vi "Volt Reader Trigger10.vi"() -> ()   [LabVIEW 2014]
uses:
  Enum State Machine Typedef.ctl
  <vilib>/Utility/error.llb/DialogType.ctl
  <vilib>/_DAQmxBase/Internals/DAQmxBase Create Channel (AI-Voltage-Basic).vi
  <vilib>/_DAQmxBase/Internals/DAQmxBase Timing (Sample Clock).vi
  <vilib>/measure/mamon.llb/Trigger Detection for 1 Channel.vi
  <vilib>/_DAQmxBase/Internals/DAQmxBase Read (Analog 2D DBL NChan NSamp).vi
  <vilib>/measure/NI_MAPro.lvlib
panel:
  out "Waveform Raw":waveform(dbl)(graph)
  in  "Offset (percent of buffer)":dbl(knob) scale=-50.0..50.0
  in  "Timeout (in iterations)":i16
  out "State":T1
  out "Waveform Graph":waveform(dbl)(graph)
  in  "Buffer (Seconds)":dbl
  out "Threshold":dbl
  in  "units":i32(ring)=10348 items=["Volts"=10348, "From Custom Scale"=10065]
  in  "stop":bool
  in  "physical channels":tag
  in  "maximum value":dbl=5.0 format="%0.2f"
  in  "minimum value":dbl=-5.0 format="%0.2f"
  in  "rate":i32=1000 caption="Sample Rate"
  # "The inputs above MUST BE\nPreset before running"
  # "NOTE: Just change the Y axis value"
  # "Make Sure that Buffer does not equal 0"
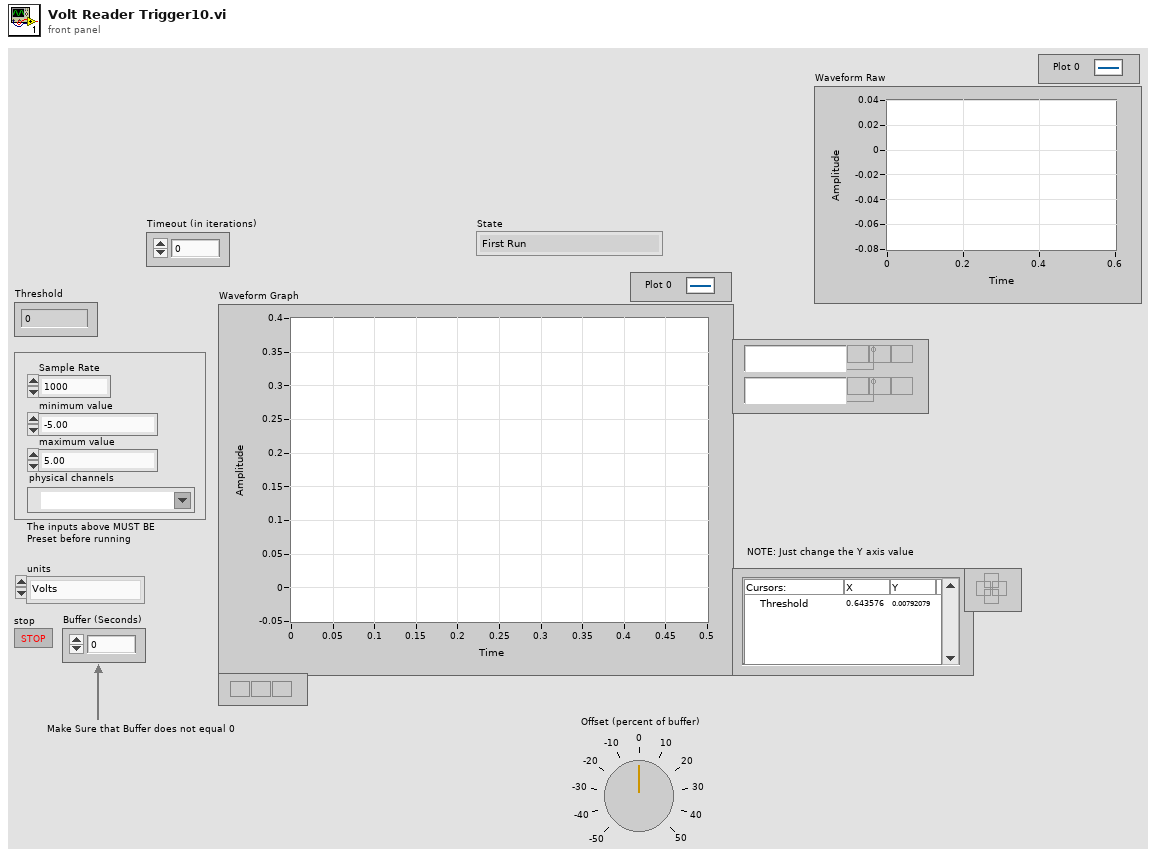
[diagram p1: front panel]
types:
  T1 = typedef "Enum State Machine Typedef.ctl" = enum16{"First Run", "Gather and Edit Data", "Find Max with Gather Data", "Trigger Occured", "Found the Max", "Just Displayed", "The Max is in the Middle", "Base State", "Timeout"}
  T2 = typedef "DialogType.ctl" = u16
  T3 = typedef "LVCursorListTypeDef.ctl" = cluster{"Name":string, "Color":u32, "Style":u8, "Point Style":u8, "Name Visible":bool, "Allow Drag":bool, "Cursor Mode":u32, "Plot":i32, "Index":i32, "Position":cluster{"X":dbl, "Y":dbl}, "X Scale":u32, "Y Scale":u32, "Watch Plots":i32[], "Watch All Plots":bool, "Plot Area":i32, "Label Offset":cluster{"X":dbl, "Y":dbl}}[]
  T4 = cluster{"Name":string, "Color":u32, "Style":u8, "Point Style":u8, "Name Visible":bool, "Allow Drag":bool, "Cursor Mode":u32, "Plot":i32, "Index":i32, "Position":cluster{"X":dbl, "Y":dbl}, "X Scale":u32, "Y Scale":u32, "Watch Plots":i32[], "Watch All Plots":bool, "Plot Area":i32, "Label Offset":cluster{"X":dbl, "Y":dbl}}
  T5 = enum16{"In the Center Range", "Before the Center Range", "After the Center Range"}
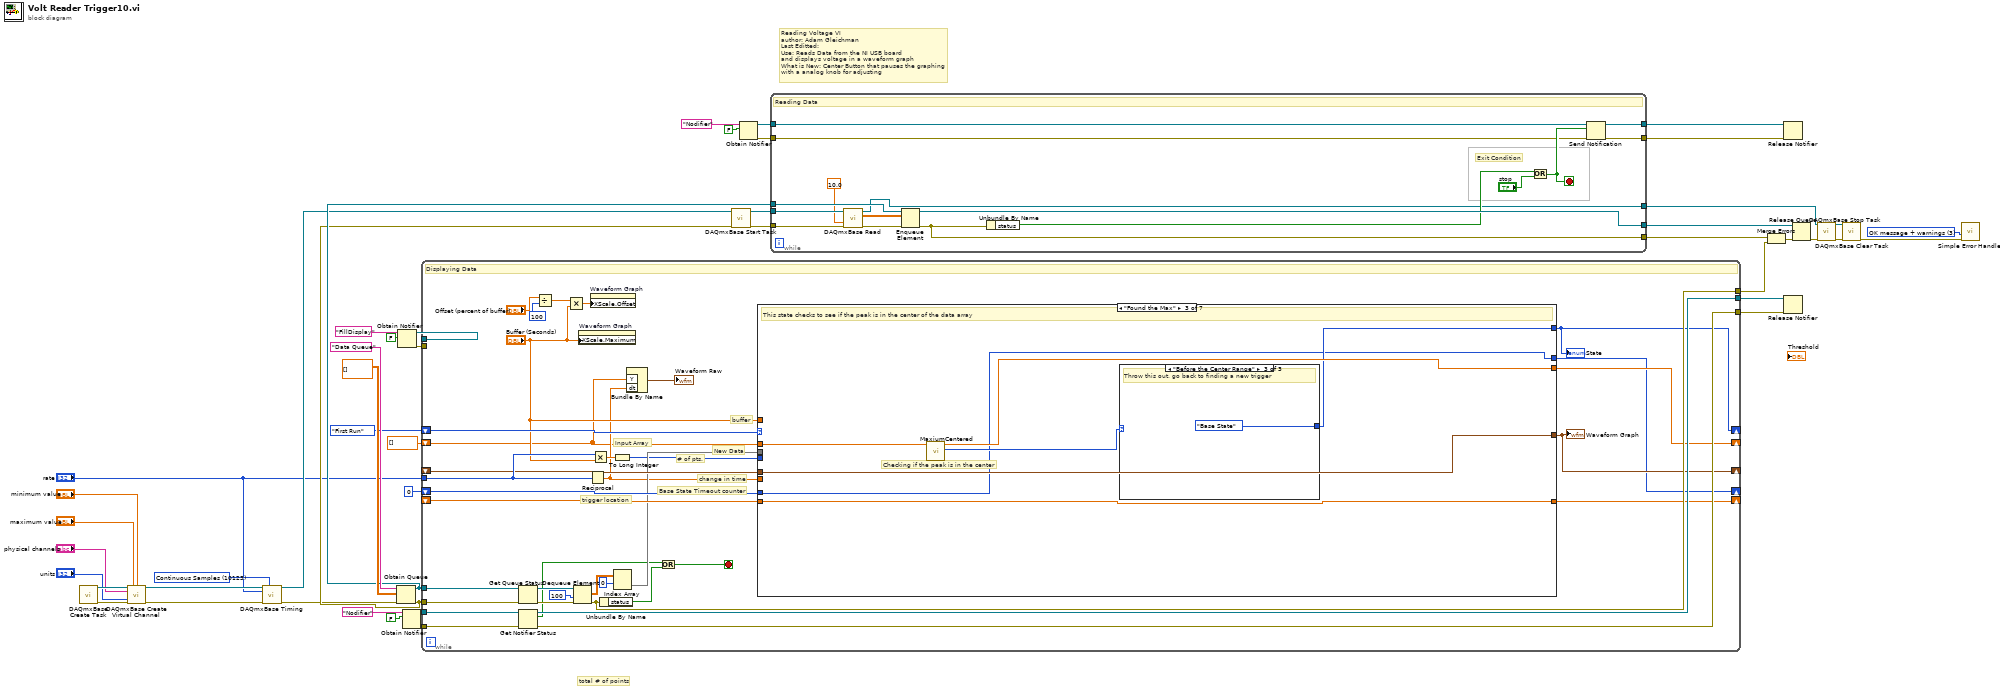
[diagram p0: block diagram]
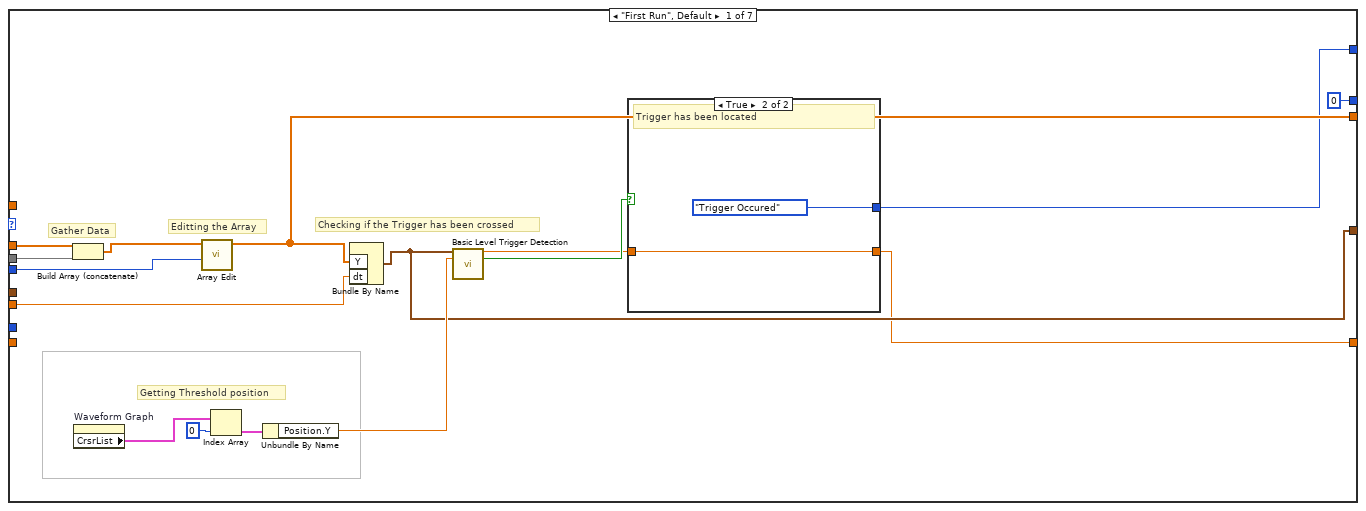
[diagram p2: hidden frame]
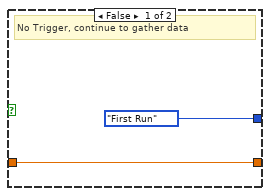
[diagram p3: hidden frame]
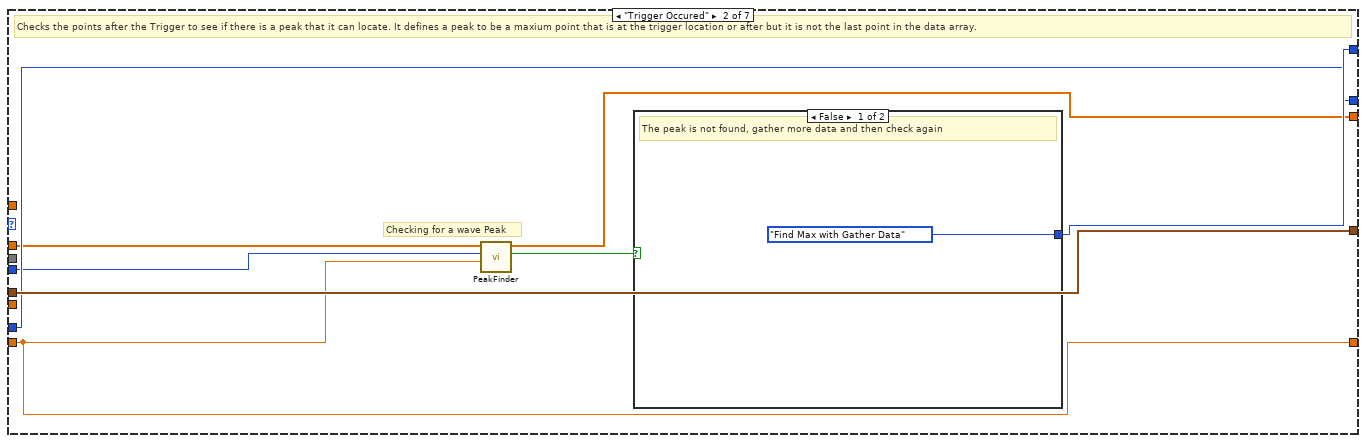
[diagram p4: hidden frame]
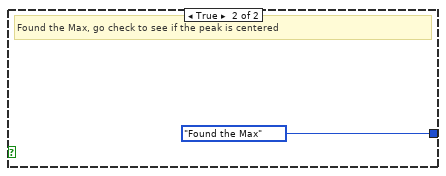
[diagram p5: hidden frame]
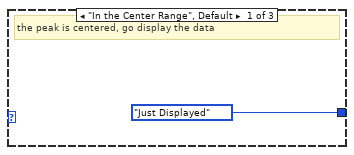
[diagram p6: hidden frame]
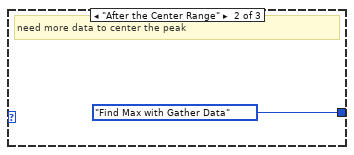
[diagram p7: hidden frame]
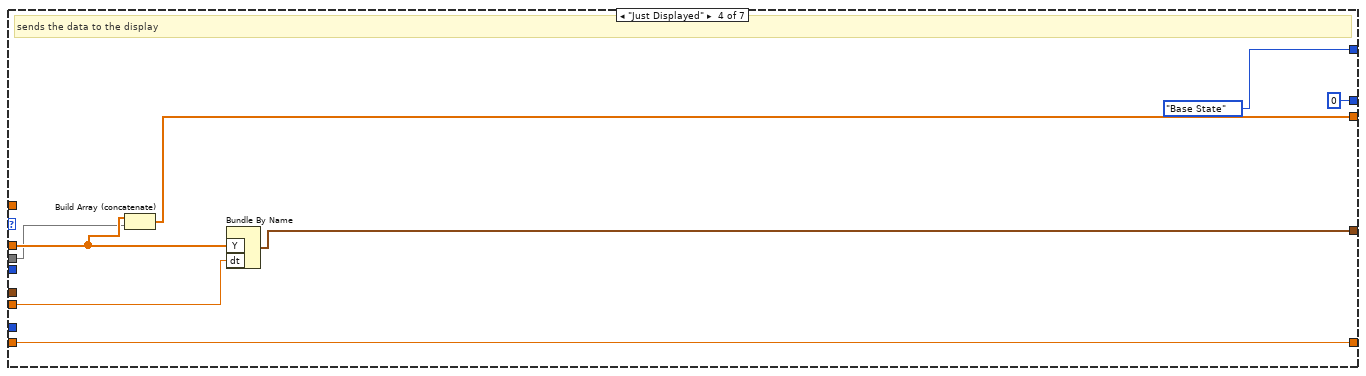
[diagram p8: hidden frame]
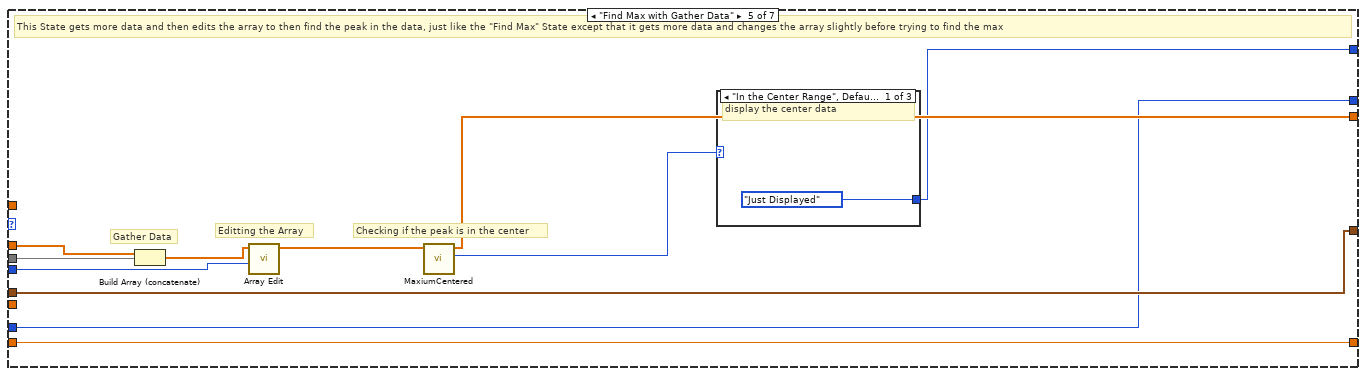
[diagram p9: hidden frame]
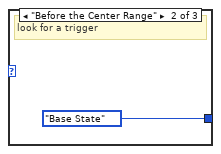
[diagram p10: hidden frame]
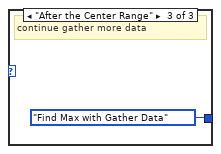
[diagram p11: hidden frame]
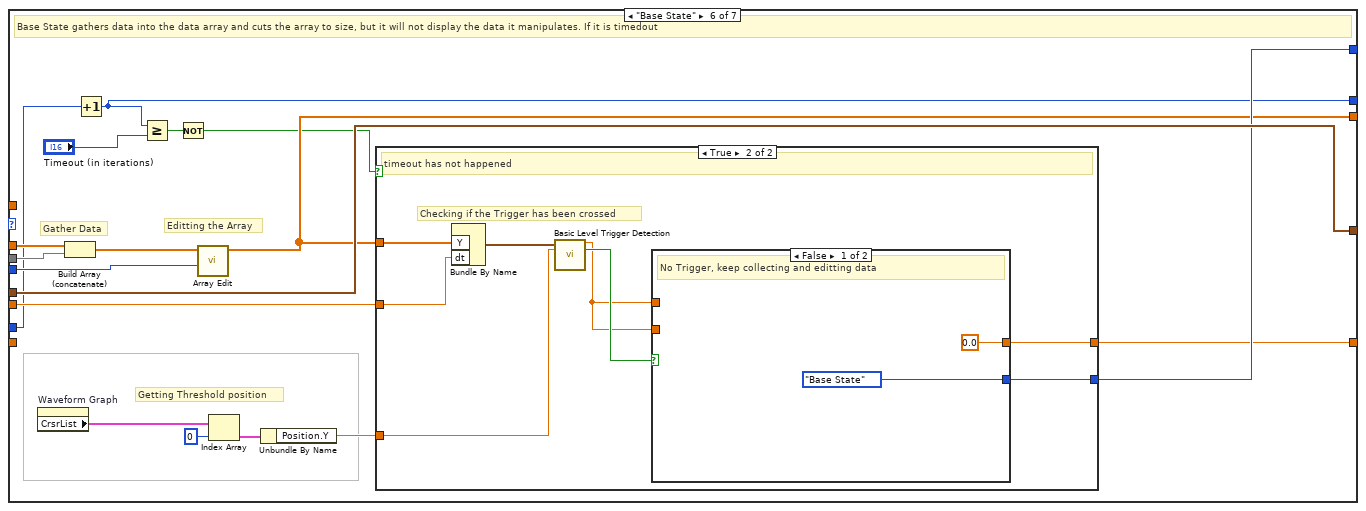
[diagram p12: hidden frame]
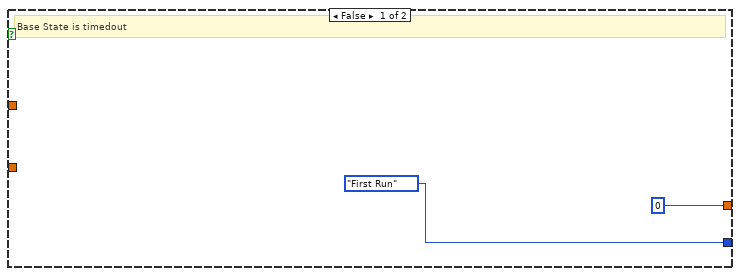
[diagram p13: hidden frame]
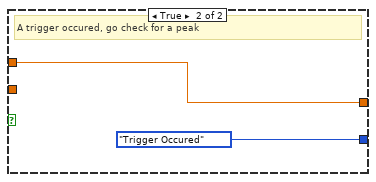
[diagram p14: hidden frame]
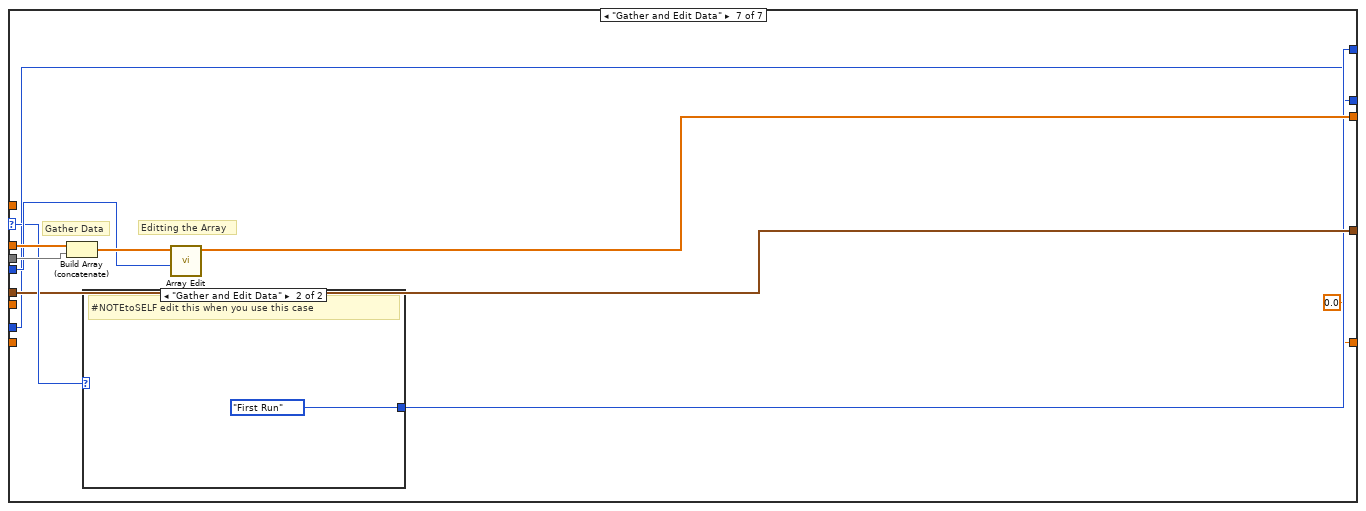
[diagram p15: hidden frame]
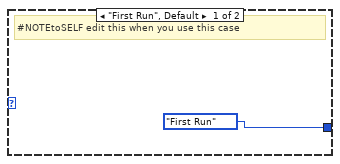
[diagram p16: hidden frame]
diagram:
  w24 = 10123 items=["Finite Samples"=10178, "Continuous Samples"=10123, "Hardware Timed Single Point"=12522] ("sample mode")
  w26 = T2 3 items=["no dialog", "OK message", "continue or stop message", "OK message + warnings", "continue/stop + warnings"] ("type of dialog (OK msg:1)")
  # "total # of points"
  # "Reading Voltage VI\nauthor: Adam Gleichman\nLast Editted: \nUse: Reads Data from the NI USB board\nand displays voltage in a waveform graph\nWhat is New: Center Button that pauses the graphing\nwith a analog knob for adjusting"
  n1 = call <vilib>:"DAQmxBase Create Task.vi"() -> ("task out"=w46:refnum<k21>, "error out"=w45:errorcluster)  [unwired: 5 in, 9 out]
  n2 = call-poly <vilib>:"DAQmxBase Create Virtual Channel.vi"("task in"=w46, "maximum value"="maximum value", "minimum value"="minimum value", "physical channels"="physical channels", "units"="units", "error in"=w45) -> ("task out"=w43:refnum<k21>, "error out"=w44:errorcluster)  [unwired: 3 in, 5 out]
  n3 = call-poly <vilib>:"DAQmxBase Timing.vi"("task/channels in"=w43, "sample mode"=w24, "rate"="rate", "error in"=w44) -> ("task out"=w12:refnum<k21>, "error out"=w11:errorcluster)  [unwired: 3 in, 7 out]
  n4 = Obtain Queue(name (unnamed)="Data Queue", element data type=dbl[][] [] ("data"), error in (no error)=w11) -> (queue out=w33:refnum<queue>, error out=w32:errorcluster)  [unwired: 2 in, 1 out]
  n5 = Obtain Notifier(name (unnamed)="FillDisplay", notification data type=FALSE) -> (notifier out=w8:refnum<notifier>, error out=w7:errorcluster)  [unwired: 2 in, 1 out]
  n6 = Obtain Notifier(name (unnamed)="Nodifier", notification data type=FALSE) -> (notifier out=w17:refnum<notifier>, error out=w15:errorcluster)  [unwired: 2 in, 1 out]
  n7 = while {
    tunnel: w33 -> [w83]
    tunnel: w32 -> [w74]
    tunnel: [w81] -> w31
    tunnel: w17 -> [w79]
    tunnel: w15 -> [w78]
    tunnel: [w77] -> w13
    tunnel: [w76] -> w14
    tunnel: "rate" -> [w70]
    shift-right: [w65] -> _
    shift-left: dbl[] [] -> [w49]
    tunnel: w8 -> [_]
    tunnel: w7 -> [_]
    shift-right: [w64] -> _
    shift-left: Enum_State_Machine_Typedef."First Run" -> [w67]
    shift-right: [w66] -> _
    shift-left: _ -> [w68]
    shift-right: [w62] -> _
    shift-left: 0 -> [w63]
    shift-right: [w61] -> _
    shift-left: _ -> [w60]
    stop <- w80 stop-if-true
    # "trigger location"
    # "change in time"
    # "buffer"
    # "Base State Timeout counter"
    # "New Data"
    # "Input Array"
    # "# of pts."
    # "Displaying Data"
    n8 = Get Queue Status(queue=w83, error in (no error)=w74) -> (queue out=w75:refnum<queue>, error out=w73:errorcluster)  [unwired: 1 in, 6 out]
    n9 = Get Notifier Status(notifier=w79, error in (no error)=w78) -> (notifier out=w77:refnum<notifier>, current notification=w51:bool, error out=w76:errorcluster)  [unwired: 2 out]
    n10 = Divide(x="Offset (percent of buffer)", y=100) -> (x/y=w54:dbl)
    n11 = Multiply(x=w54, y="Buffer (Seconds)") -> (x*y=w53:dbl)
    n12 = Dequeue Element(queue=w75, timeout in ms (-1)=100, error in (no error)=w73) -> (element=w71:dbl[][], error out=w81:errorcluster)  [unwired: 2 out]
    n13 = property on="Waveform Graph" class="WFGraph (strict)"("XScale.Maximum"="Buffer (Seconds)") -> ()  [unwired: 2 in, 2 out]
    n14 = Reciprocal(x=w70) -> (1/x=w50:dbl)
    n15 = property on="Waveform Graph" class="WFGraph (strict)"("XScale.Offset"=w53) -> ()  [unwired: 2 in, 2 out]
    n16 = Multiply(x=w70, y="Buffer (Seconds)") -> (x*y=w69:dbl)
    n17 = Unbundle By Name(w81) -> ("status"=w52:bool)
    n18 = To Long Integer(number=w69) -> (32bit integer=w58:i32)
    n19 = Index Array(array=w71, index (row)=0 ("index")) -> (element=w59:dbl[])  [unwired: 1 in]
    n20 = Bundle By Name("Y"=w49, "dt"=w50) -> (→"Waveform Raw":waveform(dbl))  [unwired: 1 in]
    n21 = Or(x=w51, y=w52) -> (x .or. y?=w80:bool)
    n22 = case shown="\"Found the Max\"" w67 {
      selector: w67 -> [_ _ _ _ _ _ w183]
      tunnel: w49 -> [w99 w108 w120 w130 w142 w163 w187]
      tunnel: w59 -> [w98 _ _ w129 w141 w162 w186]
      tunnel: w50 -> [w92 _ _ w131 _ w156 _]
      tunnel: w58 -> [w96 w105 _ _ w139 w160 w184]
      tunnel: [w89 w111 w116 w127 w134 w155 w181] -> w66
      tunnel: w68 -> [_ w111 w116 _ w134 w155 w181]
      tunnel: "Buffer (Seconds)" -> [_ _ _ _ _ _ _]
      tunnel: [w88 w107 w119 w128 w136 w153 w182] -> w65
      tunnel: [w87 w110 w117 Enum_State_Machine_Typedef."Base State" w135 w154 w180] -> w64
      tunnel: w63 -> [_ w109 w114 _ w133 w151 w179]
      tunnel: [0 w109 w114 0 w133 w147 w179] -> w62
      tunnel: [w85 w104 w115 w125 w132 w146 0.0 ("trigger location")] -> w61
      tunnel: w60 -> [_ w104 w115 w125 w132 _ _]
      frame "First Run", Default {
        # "Checking if the Trigger has been crossed"
        # "Getting Threshold position"
        # "Editting the Array"
        # "Gather Data"
        n23 = Build Array (concatenate)(w99, w98) -> (w97:dbl[])
        n24 = property on="Waveform Graph" class="WFGraph (strict)"() -> ("CrsrList"=w94:T3)  [unwired: 2 in, 2 out]
        n25 = call "Array Edit.vi"("Number of Points"=w96, "Y-values"=w97) -> ("Editted Y Values"=w88:dbl[])  [unwired: 9 in]
        n26 = Index Array(array=w94, index=0) -> (element=w95:T4)
        n27 = Unbundle By Name(w95) -> ("Position.Y"=w91:dbl)
        n28 = Bundle By Name("Y"=w88, "dt"=w92) -> (w89:waveform(dbl))  [unwired: 1 in]
        n29 = call-poly <vilib>:"Basic Level Trigger Detection.vi"("signal in"=w89, "level"=w91) -> ("trigger location"=w86:dbl, "trigger detected?"=w90:bool)  [unwired: 11 in, 1 out]
        n30 = case shown="True" w90 {
          tunnel: [Enum_State_Machine_Typedef."First Run" Enum_State_Machine_Typedef."Trigger Occured"] -> w87
          tunnel: w86 -> [w100 w102]
          tunnel: [w100 w102] -> w85
          frame False {
            # "No Trigger, continue to gather data"
          }
          frame True {
            # "Trigger has been located"
          }
        }
      }
      frame "Trigger Occured" {
        # "Checking for a wave Peak"
        # "Checks the points after the Trigger to see if there is a peak that it can locate. It defines a peak to be a maxium point that is at the trigger location or after but it is not the last point in the data array."
        n31 = call "PeakFinder.vi"("Trigger location"=w104, "Number of Points"=w105, "Input Y values"=w108) -> ("peak?"=w106:bool, "Input Y values"=w107:dbl[])  [unwired: 7 in]
        n32 = case shown="False" w106 {
          tunnel: [Enum_State_Machine_Typedef."Find Max with Gather Data" Enum_State_Machine_Typedef."Found the Max"] -> w110
          frame False {
            # "The peak is not found, gather more data and then check again"
          }
          frame True {
            # "Found the Max, go check to see if the peak is centered"
          }
        }
      }
      frame "Found the Max" {
        # "Checking if the peak is in the center"
        # "This state checks to see if the peak is in the center of the data array"
        n33 = call "MaxiumCentered.vi"("Input Y Values"=w120) -> ("State output"=w118:T5, "Output Y Values"=w119:dbl[])  [unwired: 9 in]
        n34 = case shown="\"Before the Center Range\"" w118 {
          tunnel: [Enum_State_Machine_Typedef."Just Displayed" Enum_State_Machine_Typedef."Find Max with Gather Data" Enum_State_Machine_Typedef."Base State"] -> w117
          frame "In the Center Range", Default {
            # "the peak is centered, go display the data"
          }
          frame "After the Center Range" {
            # "need more data to center the peak"
          }
          frame "Before the Center Range" {
            # "Throw this out, go back to finding a new trigger"
          }
        }
      }
      frame "Just Displayed" {
        # "sends the data to the display"
        n35 = Build Array (concatenate)(w130, w129) -> (w128:dbl[])
        n36 = Bundle By Name("Y"=w130, "dt"=w131) -> (w127:waveform(dbl))  [unwired: 1 in]
      }
      frame "Find Max with Gather Data" {
        # "Editting the Array"
        # "Gather Data"
        # "Checking if the peak is in the center"
        # "This State gets more data and then edits the array to then find the peak in the data, just like the \"Find Max\" State except that it gets more data and changes the array slightly before trying to find the max"
        n37 = Build Array (concatenate)(w142, w141) -> (w140:dbl[])
        n38 = call "Array Edit.vi"("Number of Points"=w139, "Y-values"=w140) -> ("Editted Y Values"=w138:dbl[])  [unwired: 9 in]
        n39 = call "MaxiumCentered.vi"("Input Y Values"=w138) -> ("State output"=w137:T5, "Output Y Values"=w136:dbl[])  [unwired: 9 in]
        n40 = case shown="\"In the Center Range\", Default" w137 {
          tunnel: [Enum_State_Machine_Typedef."Just Displayed" Enum_State_Machine_Typedef."Base State" Enum_State_Machine_Typedef."Find Max with Gather Data"] -> w135
          frame "In the Center Range", Default {
            # "display the center data"
          }
          frame "Before the Center Range" {
            # "look for a trigger"
          }
          frame "After the Center Range" {
            # "continue gather more data"
          }
        }
      }
      frame "Base State" {
        # "Getting Threshold position"
        # "Editting the Array"
        # "Gather Data"
        # "Base State gathers data into the data array and cuts the array to size, but it will not display the data it manipulates. If it is timedout"
        n41 = property on="Waveform Graph" class="WFGraph (strict)"() -> ("CrsrList"=w152:T3)  [unwired: 2 in, 2 out]
        n42 = Build Array (concatenate)(w163, w162) -> (w161:dbl[])
        n43 = Increment(x=w151) -> (x+1=w147:i32)
        n44 = Greater Or Equal?(x=w147, y="Timeout (in iterations)") -> (x >= y?=w149:bool)
        n45 = Not(x=w149) -> (.not. x?=w148:bool)
        n46 = call "Array Edit.vi"("Number of Points"=w160, "Y-values"=w161) -> ("Editted Y Values"=w153:dbl[])  [unwired: 9 in]
        n47 = Index Array(array=w152, index=0) -> (element=w159:T4)
        n48 = Unbundle By Name(w159) -> ("Position.Y"=w157:dbl)
        n49 = case shown="True" w148 {
          tunnel: w157 -> [_ w172]
          tunnel: w156 -> [_ w171]
          tunnel: [Enum_State_Machine_Typedef."First Run" w169] -> w154
          tunnel: w153 -> [_ w168]
          tunnel: [0 w166] -> w146
          frame False {
            # "Base State is timedout"
          }
          frame True {
            # "Checking if the Trigger has been crossed"
            # "timeout has not happened"
            n50 = Bundle By Name("Y"=w168, "dt"=w171) -> (w173:waveform(dbl))  [unwired: 1 in]
            n51 = call-poly <vilib>:"Basic Level Trigger Detection.vi"("signal in"=w173, "level"=w172) -> ("trigger location"=w167:dbl, "trigger detected?"=w170:bool)  [unwired: 11 in, 1 out]
            n52 = case shown="False" w170 {
              tunnel: [Enum_State_Machine_Typedef."Base State" Enum_State_Machine_Typedef."Trigger Occured"] -> w169
              tunnel: w167 -> [_ _]
              tunnel: [0.0 w176] -> w166
              tunnel: w167 -> [_ w176]
              frame False {
                # "No Trigger, keep collecting and editting data"
              }
              frame True {
                # "A trigger occured, go check for a peak"
              }
            }
          }
        }
      }
      frame "Gather and Edit Data" {
        # "Editting the Array"
        # "Gather Data"
        n53 = Build Array (concatenate)(w187, w186) -> (w185:dbl[])
        n54 = case shown="\"Gather and Edit Data\"" w183 {
          tunnel: [Enum_State_Machine_Typedef."First Run" Enum_State_Machine_Typedef."First Run"] -> w180
          frame "First Run", Default {
            # "#NOTEtoSELF edit this when you use this case"
          }
          frame "Gather and Edit Data" {
            # "#NOTEtoSELF edit this when you use this case"
          }
        }
        n55 = call "Array Edit.vi"("Number of Points"=w184, "Y-values"=w185) -> ("Editted Y Values"=w182:dbl[])  [unwired: 9 in]
      }
    }
    "Waveform Graph" <- w66
    "State" <- w64
  }
  n56 = call <vilib>:"DAQmxBase Start Task.vi"("task/channels in"=w12, "error in"=w32) -> ("task out"=w41:refnum<k21>, "error out"=w42:errorcluster)  [unwired: 12 out]
  n57 = Obtain Notifier(name (unnamed)="Nodifier", notification data type=FALSE) -> (notifier out=w20:refnum<notifier>, error out=w19:errorcluster)  [unwired: 2 in, 1 out]
  n58 = while "Data Reading Loop" {
    tunnel: w42 -> [w204]
    tunnel: w41 -> [w205]
    tunnel: w33 -> [w202]
    tunnel: [w199] -> w36
    tunnel: [w197] -> w35
    tunnel: [w195] -> w23
    tunnel: w20 -> [w193]
    tunnel: w19 -> [w192]
    tunnel: [w191] -> w10
    tunnel: [w190] -> w9
    stop <- w194 stop-if-true
    # "Exit Condition"
    # "Reading Data"
    n59 = call-poly <vilib>:"DAQmxBase Read.vi"("task/channels in"=w205, "timeout"=10.0, "error in"=w204) -> ("task out"=w195:refnum<k21>, "data"=w200:dbl[][], "error out"=w203:errorcluster)  [unwired: 10 in]
    n60 = Enqueue Element(queue=w202, element=w200, error in (no error)=w203) -> (queue out=w199:refnum<queue>, error out=w197:errorcluster)  [unwired: 1 in, 1 out]
    n61 = Unbundle By Name(w197) -> ("status"=w196:bool)
    n62 = Or(x=w196, y="stop") -> (x .or. y?=w194:bool)
    n63 = Send Notification(notification=w194, notifier=w193, error in (no error)=w192) -> (notifier out=w191:refnum<notifier>, error out=w190:errorcluster)
  }
  n64 = Merge Errors(w35, w31) -> (w34:errorcluster)
  n65 = Release Notifier(notifier=w10, error in (no error)=w9) -> ()  [unwired: 1 in, 3 out]
  n66 = Release Notifier(notifier=w13, error in (no error)=w14) -> ()  [unwired: 1 in, 3 out]
  n67 = Release Queue(queue=w36, error in (no error)=w34) -> (error out=w30:errorcluster)  [unwired: 1 in, 2 out]
  n68 = call <vilib>:"DAQmxBase Stop Task.vi"("task/channels in"=w23, "error in"=w30) -> ("task out"=w29:refnum<k21>, "error out"=w28:errorcluster)  [unwired: 12 in]
  n69 = call <vilib>:"DAQmxBase Clear Task.vi"("task in"=w29, "error in"=w28) -> ("error out"=w27:errorcluster)  [unwired: 13 in]
  n70 = call <vilib>:"Simple Error Handler.vi"("type of dialog (OK msg:1)"=w26, "error in (no error)"=w27) -> ()  [unwired: 3 in, 5 out]
